vi "GetContMeasData.vi"(8 "error in (no error)":errorcluster, 11 "TCP Network Connection in":refnum<k5>) -> (0 "error out":errorcluster, 2 "Meas Result":dbl[](array[numeric]), 3 "TCP Network Connection out":refnum<k5>, 5 "Sonstige Nachrichten":string[](array[string]))   [LabVIEW 2017]
uses:
  AT901 API/TypeDefinitions/ES_DataType.ctl
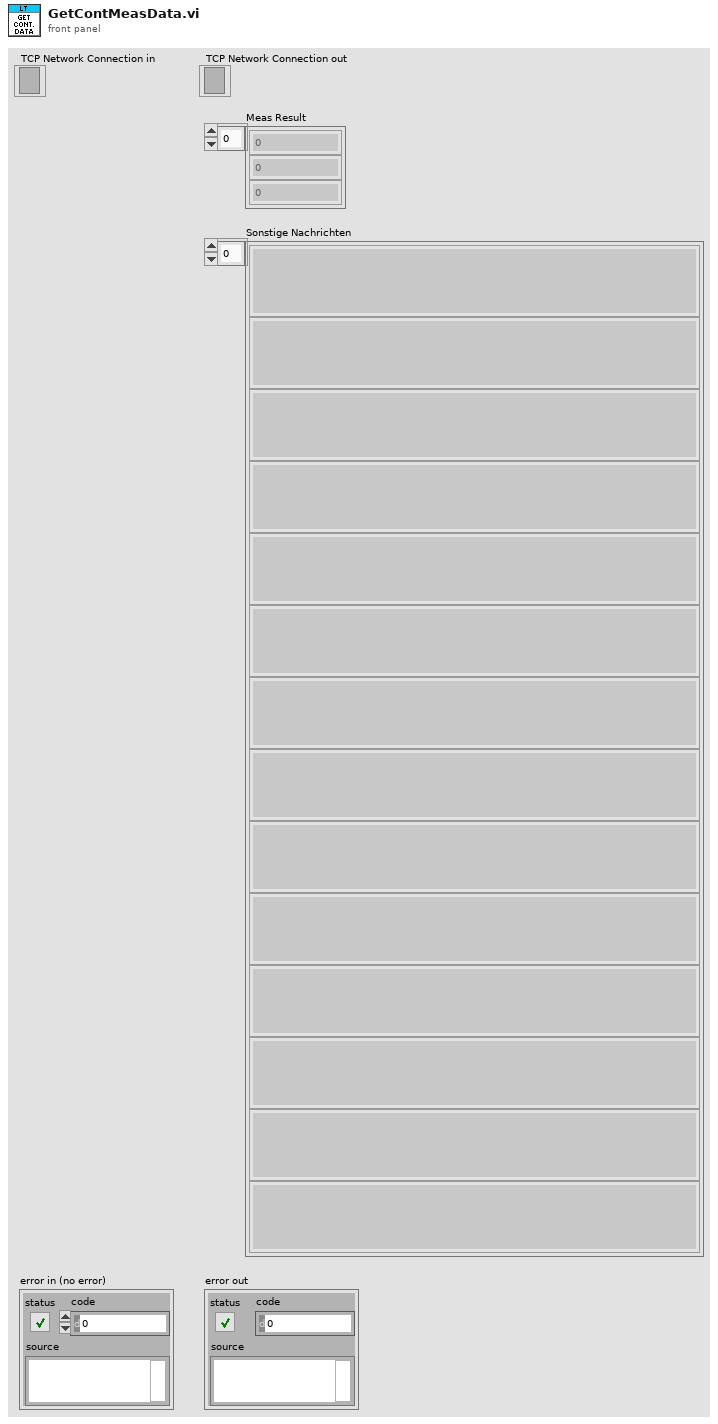
[diagram p1: front panel]
types:
  T1 = typedef "ES_DataType.ctl" = enum32{"ES_DT_Command", "ES_DT_Error", "ES_DT_SingleMeasResult", "ES_DT_MultiMeasResult", "ES_DT_StationaryProbeMeasResult", "ES_DT_ContinuousProbeMeasResult", "ES_DT_NivelResult", "ES_DT_ReflectorPosResult", "ES_DT_SystemStatusChange", "ES_DT_SingleMeasResult2", "ES_DT_MultiMeasResult2", "ES_DT_ProbePosResult"}
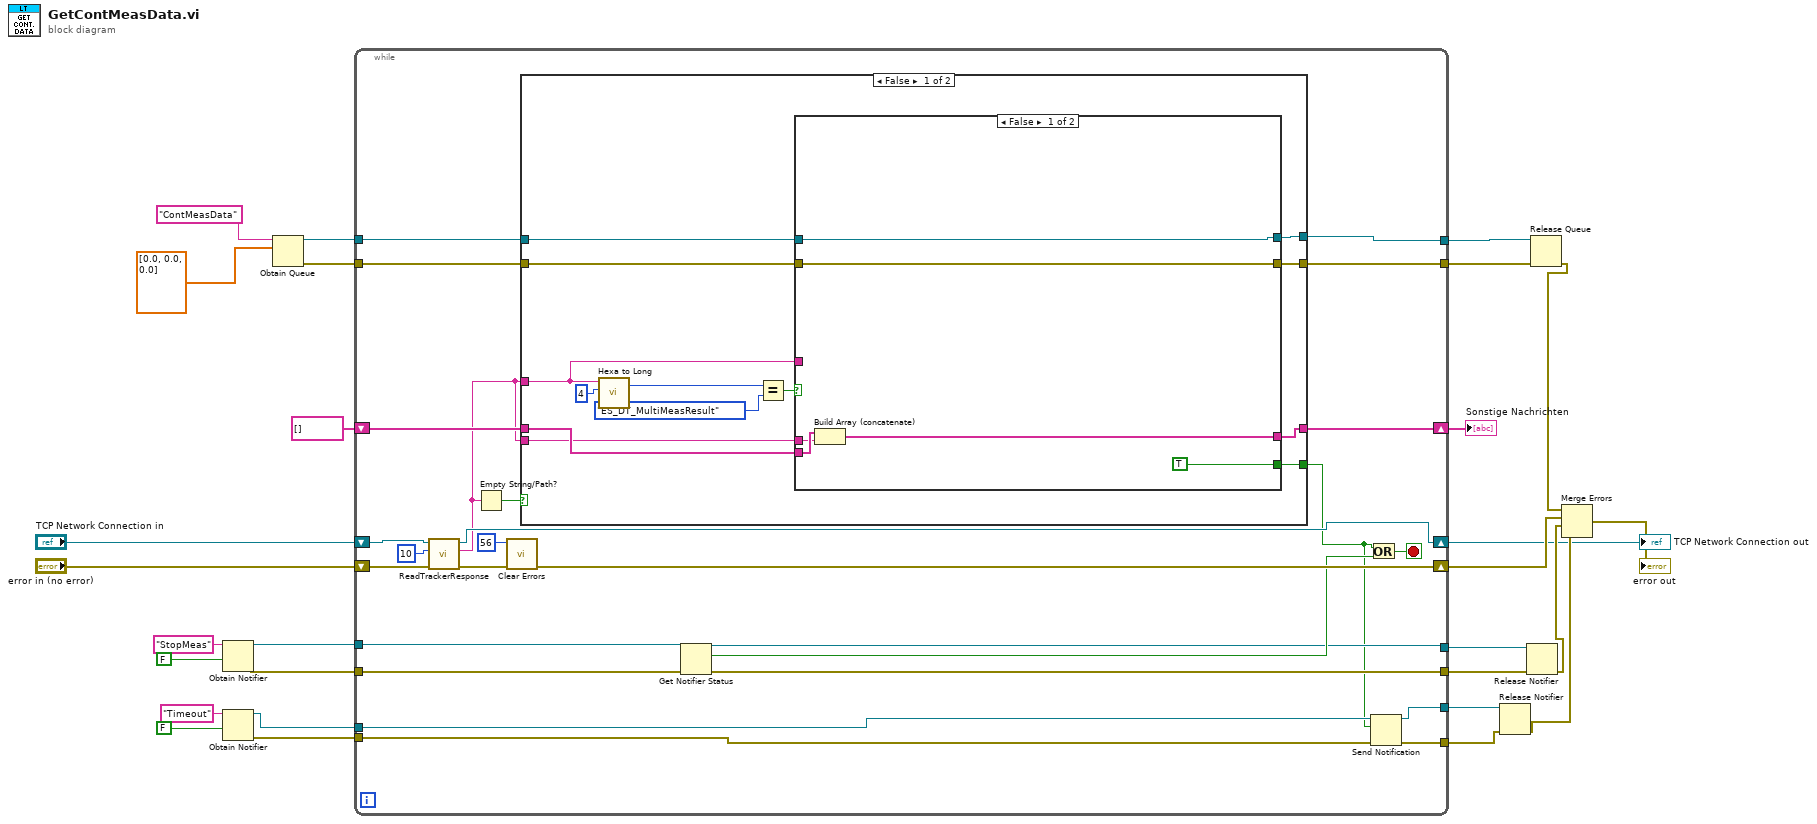
[diagram p0: block diagram]
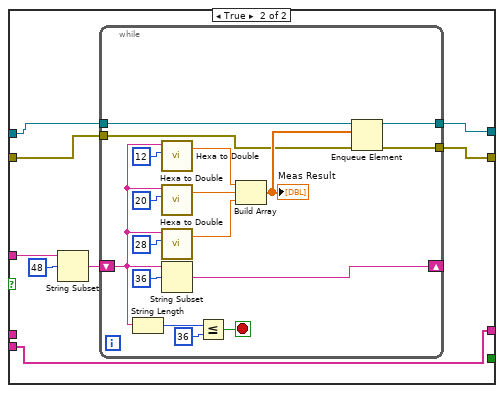
[diagram p2: hidden frame]
diagram:
  n1 = Obtain Notifier(name (unnamed)="StopMeas", notification data type=FALSE) -> (notifier out=w13:refnum<notifier>, error out=w12:errorcluster)  [unwired: 2 in, 1 out]
  n2 = Obtain Notifier(name (unnamed)="Timeout", notification data type=FALSE) -> (notifier out=w20:refnum<notifier>, error out=w21:errorcluster)  [unwired: 2 in, 1 out]
  n3 = Obtain Queue(name (unnamed)="ContMeasData", element data type=dbl[] [0.0, 0.0, 0.0] ("Meas Result")) -> (queue out=w8:refnum<queue>, error out=w9:errorcluster)  [unwired: 3 in, 1 out]
  n4 = while {
    shift-right: [w53] -> w5
    shift-left: "TCP Network Connection in" -> [w54]
    shift-right: [w49] -> w25
    shift-left: "error in (no error)" -> [w52]
    shift-right: [w44] -> w4
    shift-left: string[] [] -> [w46]
    tunnel: w8 -> [w42]
    tunnel: w9 -> [w41]
    tunnel: [w40] -> w11
    tunnel: [w39] -> w10
    tunnel: w12 -> [w38]
    tunnel: w13 -> [w37]
    tunnel: [w34] -> w15
    tunnel: [w35] -> w16
    tunnel: w20 -> [w33]
    tunnel: w21 -> [w32]
    tunnel: [w30] -> w22
    tunnel: [w29] -> w23
    stop <- w43 stop-if-true
    n5 = call "ReadTrackerResponse.vi"("error in"=w52, "timeout ms (1000)"=10, "connection ID in"=w54) -> ("error out"=w50:errorcluster, "Tracker Response"=w45:string, "connection ID out"=w53:refnum<k5>)  [unwired: 6 in]
    n6 = Empty String/Path?(string/path=w45) -> (empty?=w47:bool)
    n7 = call <vilib>:"Clear Errors.vi"("error in (no error)"=w50, "specific error code to clear (0: all)"=56) -> ("error out"=w49:errorcluster)  [unwired: 4 in, 1 out]
    n8 = case shown="False" w47 {
      tunnel: w45 -> [w63 _]
      tunnel: w46 -> [w62 w101]
      tunnel: w45 -> [w61 _]
      tunnel: [w60 w101] -> w44
      tunnel: [w59 _] -> w31
      tunnel: w42 -> [w58 w100]
      tunnel: w41 -> [w57 w99]
      tunnel: [w56 w99] -> w40
      tunnel: [w55 w100] -> w39
      frame False {
        n9 = call "Hexa to Long.vi"("Hexa"=w63, "Index"=4) -> ("Long"=w66:u32)  [unwired: 4 in]
        n10 = Equal?(x=w66, y=ES_DataType."ES_DT_MultiMeasResult" ("ES_DataType")) -> (x = y?=w64:bool)
        n11 = case shown="False" w64 {
          tunnel: w63 -> [_ w79]
          tunnel: w62 -> [w73 w78]
          tunnel: w61 -> [w72 _]
          tunnel: [w71 w78] -> w60
          tunnel: [TRUE _] -> w59
          tunnel: w58 -> [w69 w77]
          tunnel: w57 -> [w68 w76]
          tunnel: [w68 w75] -> w56
          tunnel: [w69 w74] -> w55
          frame False {
            n12 = Build Array (concatenate)(w73, w72) -> (w71:string[])
          }
          frame True {
            n13 = String Subset(string=w79, offset (0)=48) -> (substring=w80:string)  [unwired: 1 in]
            n14 = while {
              shift-right: [w87] -> _
              shift-left: w80 -> [w88]
              tunnel: w77 -> [w85]
              tunnel: w76 -> [w84]
              tunnel: [w83] -> w75
              tunnel: [w82] -> w74
              stop <- w96 stop-if-true
              n15 = String Length(string=w88) -> (length=w98:i32)
              n16 = call "Hexa to Double.vi"("Hexa"=w88, "Index"=12) -> ("Double"=w95:dbl)  [unwired: 4 in]
              n17 = call "Hexa to Double.vi"("Hexa"=w88, "Index"=20) -> ("Double"=w94:dbl)  [unwired: 4 in]
              n18 = call "Hexa to Double.vi"("Hexa"=w88, "Index"=28) -> ("Double"=w93:dbl)  [unwired: 4 in]
              n19 = String Subset(string=w88, offset (0)=36) -> (substring=w87:string)  [unwired: 1 in]
              n20 = Less Or Equal?(x=w98, y=36) -> (x <= y?=w96:bool)
              n21 = Build Array(w95, w94, w93) -> (w86:dbl[])
              "Meas Result" <- w86
              n22 = Enqueue Element(queue=w85, element=w86, error in (no error)=w84) -> (queue out=w82:refnum<queue>, error out=w83:errorcluster)  [unwired: 1 in, 1 out]
            }
          }
        }
      }
      frame True {
      }
    }
    n23 = Get Notifier Status(notifier=w37, error in (no error)=w38) -> (notifier out=w34:refnum<notifier>, current notification=w36:bool, error out=w35:errorcluster)  [unwired: 2 out]
    n24 = Or(x=w31, y=w36) -> (x .or. y?=w43:bool)
    n25 = Send Notification(notification=w31, notifier=w33, error in (no error)=w32) -> (notifier out=w30:refnum<notifier>, error out=w29:errorcluster)
  }
  "Sonstige Nachrichten" <- w4
  "TCP Network Connection out" <- w5
  n26 = Release Notifier(notifier=w22, error in (no error)=w23) -> (error out=w27:errorcluster)  [unwired: 1 in, 2 out]
  n27 = Release Notifier(notifier=w15, error in (no error)=w16) -> (error out=w26:errorcluster)  [unwired: 1 in, 2 out]
  n28 = Release Queue(queue=w10, error in (no error)=w11) -> (error out=w24:errorcluster)  [unwired: 1 in, 2 out]
  n29 = Merge Errors(w24, w25, w26, w27) -> (→"error out":errorcluster)
